vi "Update Acquisition Hold-Off Points in Record.vi"(8 "Increment?":bool, 9 "Trigger Hold Off Ticks Finished":u16, 11 "Trigger Hold-Off Ticks":u16) -> (0 "Trigger Hold Off Ticks Finish":bool, 1 "Updated Trigger Hold Off Done":u16, 2 "Is Trigger Hold Off =0?":bool)   [LabVIEW 2012]
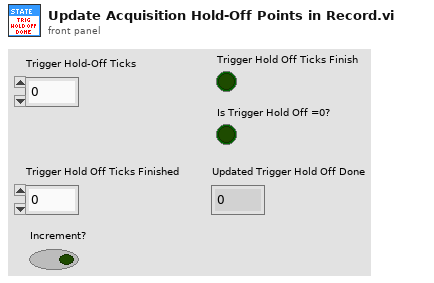
[diagram p1: front panel]
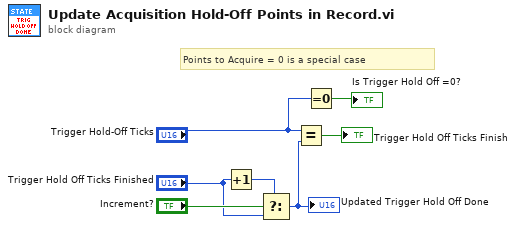
[diagram p0: block diagram]
diagram:
  # "Points to Acquire = 0 is a special case"
  n1 = Increment(x="Trigger Hold Off Ticks Finished") -> (x+1=w7:u16)
  n2 = Select(t=w7, s="Increment?", f="Trigger Hold Off Ticks Finished") -> (s? t:f=w4:u16)
  "Updated Trigger Hold Off Done" <- w4
  n3 = Equal?(x="Trigger Hold-Off Ticks", y=w4) -> (x = y?=→"Trigger Hold Off Ticks Finish":bool)
  n4 = Equal To 0?(x="Trigger Hold-Off Ticks") -> (x = 0?=→"Is Trigger Hold Off =0?":bool)
